vi "ObservadorPerturbacion.vi"(0 "entrada planta":dbl, 8 "salida planta":dbl, 11 "xk +1":T1=[[0.0], [0.0]]) -> (1 "Perturbacion":dbl, 3 "xk":T1)   [LabVIEW 2018]
uses:
  <vilib>/Analysis/Matrix/Datatypes/RealMatrix.ctl
  <vilib>/Analysis/Matrix/Numeric/Conversions/Array To Matrix - RA.vi
  <vilib>/Analysis/Matrix/Numeric/Conversions/Array To Matrix - RA2.vi
  <vilib>/Analysis/Matrix/Numeric/Multiply/Multiply - RM,RM.vi
  <vilib>/Analysis/Matrix/Numeric/Add/Add - RM,RM.vi
  <vilib>/Analysis/Matrix/NI_Matrix.lvlib
panel:
  out "A + B":T1
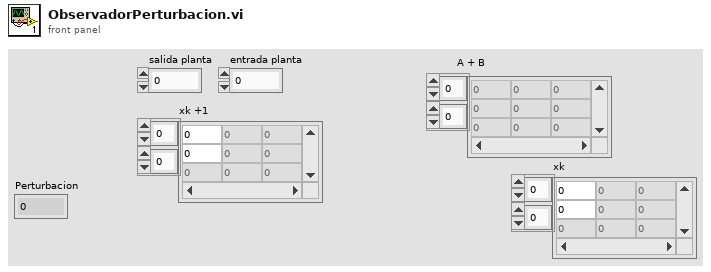
[diagram p1: front panel]
types:
  T1 = typedef "NI_Matrix.lvlib/RealMatrix.ctl" = dbl[][]
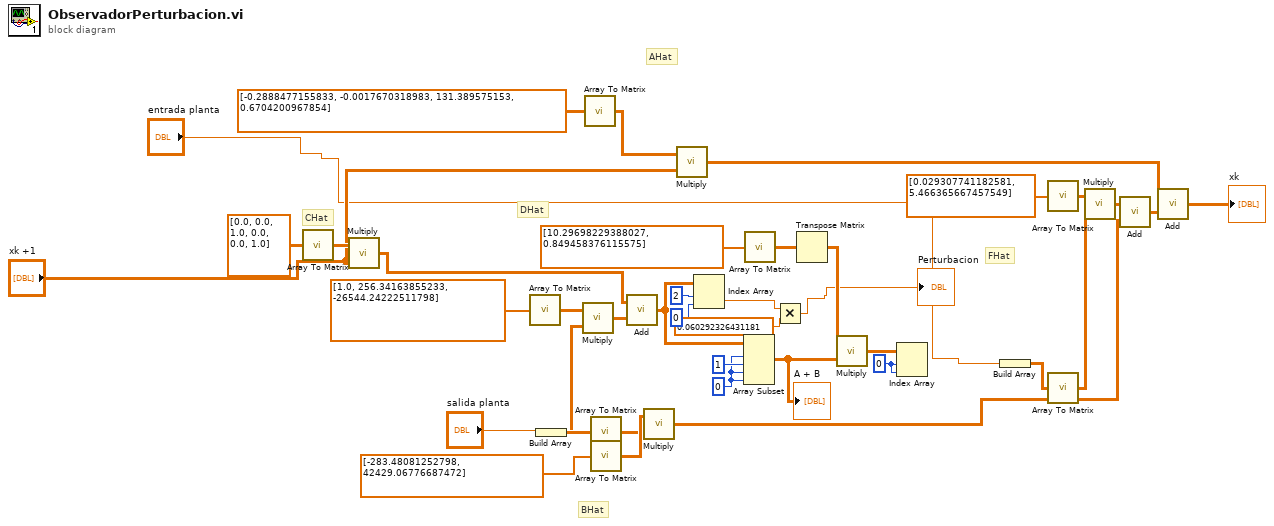
[diagram p0: block diagram]
diagram:
  w33 = 0 ("index (row)")
  w35 = 0 ("row 1")
  # "DHat"
  # "CHat"
  # "FHat"
  # "AHat"
  # "BHat"
  n1 = call-poly <vilib>:"Array To Matrix.vi"("Real 2D Array"=dbl[][] [[0.0, 0.0], [1.0, 0.0], [0.0, 1.0]]) -> ("Real Matrix"=w16:T1)
  n2 = call-poly <vilib>:"Multiply.vi"("Real Matrix B"="xk +1", "Real Matrix A"=w16) -> ("A * B"=w15:T1)
  n3 = call-poly <vilib>:"Array To Matrix.vi"("Real 1D Array"=dbl[] [1.0, 256.34163855233, -26544.24222511798] ("element")) -> ("Real Matrix (Column Vector)"=w26:T1)
  n4 = Build Array("salida planta") -> (w37:T1)
  n5 = call-poly <vilib>:"Array To Matrix.vi"("Real 2D Array"=dbl[][] [[-0.2888477155833, -0.0017670318983], [131.389575153, 0.6704200967854]] ("element")) -> ("Real Matrix"=w25:T1)
  n6 = call-poly <vilib>:"Array To Matrix.vi"("Real 2D Array"=w37) -> ("Real Matrix"=w19:T1)
  n7 = call-poly <vilib>:"Multiply.vi"("Real Matrix B"=w19, "Real Matrix A"=w26) -> ("A * B"=w17:T1)
  n8 = call-poly <vilib>:"Array To Matrix.vi"("Real 1D Array"=dbl[] [-283.48081252798, 42429.06776687472] ("element")) -> ("Real Matrix (Column Vector)"=w20:T1)
  n9 = call-poly <vilib>:"Add.vi"("Real Matrix B"=w17, "Real Matrix A"=w15) -> ("A + B"=w10:T1)
  n10 = call-poly <vilib>:"Multiply.vi"("Real Matrix B"=w19, "Real Matrix A"=w20) -> ("A * B"=w18:T1)
  n11 = call-poly <vilib>:"Multiply.vi"("Real Matrix B"="xk +1", "Real Matrix A"=w25) -> ("A * B"=w24:T1)
  n12 = Index Array(array=w10, index (row)=2, index (col)=0) -> (element=w2:dbl)
  n13 = Array Subset(array=w10, index (row)=w35, length (row)=1 ("row N"), index (col)=w35, length (col)=w35) -> (w13:T1)
  "A + B" <- w13
  n14 = call-poly <vilib>:"Array To Matrix.vi"("Real 1D Array"=dbl[] [10.29698229388027, 0.849458376115575] ("element")) -> ("Real Matrix (Column Vector)"=w34:T1)
  n15 = Multiply(x=w2, y=0.060292326431181) -> (x*y=→"Perturbacion":dbl)
  n16 = Transpose Matrix(1:w34) -> (0:w14:T1)
  n17 = call-poly <vilib>:"Multiply.vi"("Real Matrix B"=w13, "Real Matrix A"=w14) -> ("A * B"=w12:T1)
  n18 = Index Array(array=w12, index (row)=w33, index (col)=w33) -> ()  [unwired: 1 out]
  n19 = Build Array("entrada planta") -> (w38:T1)
  n20 = call-poly <vilib>:"Array To Matrix.vi"("Real 1D Array"=dbl[] [0.029307741182581, 5.466365667457549] ("element")) -> ("Real Matrix (Column Vector)"=w23:T1)
  n21 = call-poly <vilib>:"Array To Matrix.vi"("Real 2D Array"=w38) -> ("Real Matrix"=w22:T1)
  n22 = call-poly <vilib>:"Multiply.vi"("Real Matrix B"=w22, "Real Matrix A"=w23) -> ("A * B"=w21:T1)
  n23 = call-poly <vilib>:"Add.vi"("Real Matrix B"=w18, "Real Matrix A"=w21) -> ("A + B"=w32:T1)
  n24 = call-poly <vilib>:"Add.vi"("Real Matrix B"=w32, "Real Matrix A"=w24) -> ("A + B"=→"xk":T1)
